vi "Add Resource (Generation).vi"(0 "instance":u8, 2 "gen in":refnum<class "niUSRP Tx DSP v2 FPGA.lvclass">=refnum, 3 "collection builder in":refnum<class "Collection Builder.lvclass">=refnum, 5 "rf blanking IO":refnum<k21>) -> (13 "gen out":refnum<class "niUSRP Tx DSP v2 FPGA.lvclass">, 14 "collection builder out":refnum<class "Collection Builder.lvclass">)   [LabVIEW 2023]
uses:
  <instrlib>/niUSRP/Reference FPGA/Tx DSP/niUSRP Tx DSP v2 FPGA.lvclass
  <instrlib>/niVST/Reference FPGA/FPGA/Tx DSP/niUSRP Tx DSP v2 FPGA.lvclass
  <instrlib>/_niInstr/Instruction Framework/v1/FPGA/Collection Builder/Collection Builder.lvclass
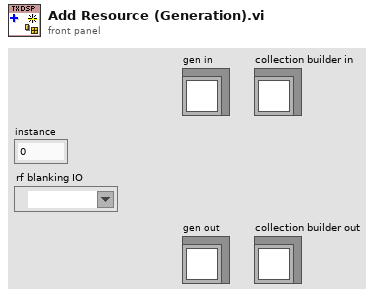
[diagram p1: front panel]
types:
  T1 = typedef "niVST Generation Registers v1 FPGA.lvclass/Generation Registers.ctl" = cluster{"dsp shared":T2}
  T2 = typedef "niVST Generation Registers v1 FPGA.lvclass/DSP Registers.ctl" = cluster{"reset":refnum<k21>, "reset.done":refnum<k21>, "ignore overflows":refnum<k21>, "overflow":refnum<k21>, "overflow.clear":refnum<k21>, "pipeline delay (pre-align)":refnum<k21>, "pipeline delay":refnum<k21>, "pipeline delay (post-align)":refnum<k21>, "group delay (output samples)":refnum<k21>, "blanking delay.data clock ticks":refnum<k21>, "dynamic delay.data clock ticks":refnum<k21>, "dynamic delay.samples":refnum<k21>, "bypass EQ":refnum<k21>, "inject idle into path":refnum<k21>}
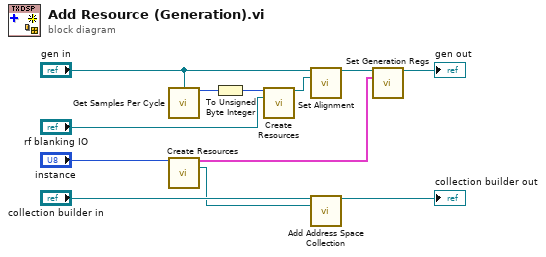
[diagram p0: block diagram]
diagram:
  n1 = call-dynamic "Get Samples Per Cycle.vi"("gen"="gen in") -> ("samples per cycle"=w2:u16)  [unwired: 14 in]
  n2 = call <instrlib>:"Create Resources.vi"("instance"="instance") -> ("gen regs"=w4:T1, "gen register collection"=w9:refnum<class "Address Space Collection.lvclass">)  [unwired: 13 in]
  n3 = To Unsigned Byte Integer(number=w2) -> (unsigned 8bit integer=w8:u8)
  n4 = call <instrlib>:"Create Resources.vi"("samples per cycle (SPC)"=w8, "rf blanking IO"="rf blanking IO") -> ("gen align"=w6:refnum<class "niVST Generation Alignment v1 FPGA.lvclass">)  [unwired: 13 in]
  n5 = call-dynamic "Set Alignment.vi"("gen in"="gen in", "align"=w6) -> ("gen out"=w7:refnum<class "niUSRP Tx DSP v2 FPGA.lvclass">)  [unwired: 13 in]
  n6 = call <instrlib>:"Add Address Space Collection.vi"("collection builder in"="collection builder in", "address space collection"=w9) -> ("collection builder out"=→"collection builder out":refnum<class "Collection Builder.lvclass">)  [unwired: 13 in]
  n7 = call-dynamic "Set Generation Regs.vi"("gen in"=w7, "gen regs"=w4) -> ("gen out"=→"gen out":refnum<class "niUSRP Tx DSP v2 FPGA.lvclass">)  [unwired: 13 in]
